vi "Send_command.vi"(9 "Команда":string, 11 "Адрес":refnum<visa-resource-name>) -> (2 "Результат":string, 3 "Адрес 2":refnum<visa-resource-name>)   [LabVIEW 2013]
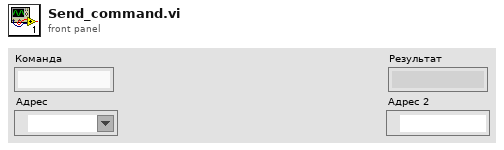
[diagram p1: front panel]
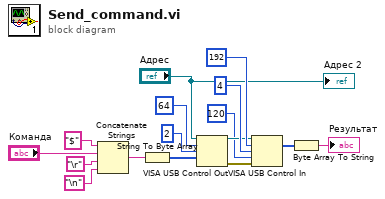
[diagram p0: block diagram]
diagram:
  n1 = Concatenate Strings("$", "Команда", "\r" ("Carriage Return"), "\n" ("Line Feed")) -> (w5:string)
  n2 = String To Byte Array(string=w5) -> (unsigned byte array=w8:u8[])
  n3 = VISA USB Control Out(0:"Адрес", 5:i16 64 ("request type"), 7:i16 2 ("request"), 9:w8) -> (4:w9:refnum<visa-resource-name>, 15:w10:errorcluster)  [unwired: 1 in, 2 out]
  n4 = VISA USB Control In(0:w9, 5:i16 192 ("request type"), 7:i16 4 ("request"), 9:u16 120 ("length (0)"), 11:w10) -> (6:w13:u8[])  [unwired: 4 out]
  n5 = Byte Array To String(unsigned byte array=w13) -> (string=→"Результат":string)
  "Адрес 2" <- "Адрес"
